vi "Wärmepumpe.ReadZustandsgrösse.vi"(0 "Wärmepumpe in":refnum<data-value>, 5 "error in":errorcluster) -> (11 "Verdichter 1":bool, 13 "Verdichter 2":bool, 14 "Wärmepumpe out":refnum<data-value>, 15 "Heizleistung [W]":dbl, 16 "Kälteleistung [W]":dbl, 17 "Vorlauftemperatur Heizkreislauf [°C]":dbl, 18 "Vorlauftemperatur Solekreislauf [°C]":dbl, 19 "error out":errorcluster)   [LabVIEW 2016, in "Wärmepumpe.lvclass"]
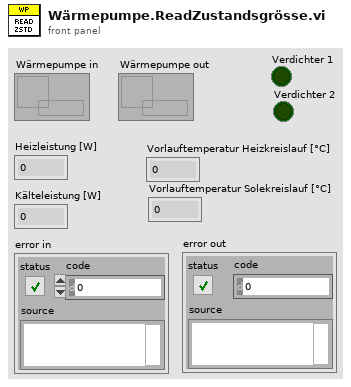
[diagram p1: front panel]
types:
  T1 = typedef "Wärmepumpe.lvclass/Wärmepumpe.Zustandsgrössen.ctl" = cluster{"Vorlauftemperatur Heizkreislauf[°C]":dbl, "Vorlauftemperatur Solekreislauf[°C]":dbl, "Heizleistung [W]":dbl, "Kälteleistung [W]":dbl, "Verdichter 1":bool, "Verdichter 2":bool}
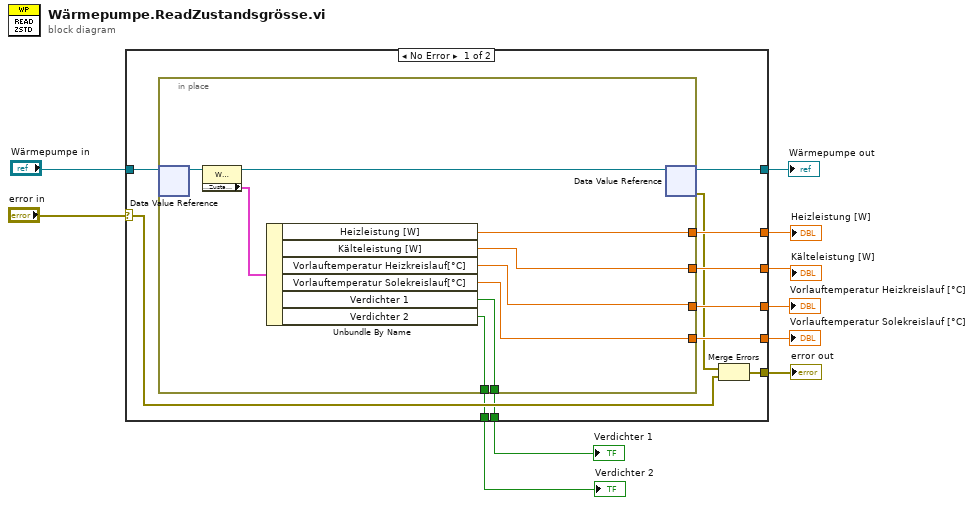
[diagram p0: block diagram]
diagram:
  n1 = case shown="No Error" "error in" {
    selector: "error in" -> [w15 w32]
    tunnel: "Wärmepumpe in" -> [w21 w31]
    tunnel: [w20 w31] -> w9
    tunnel: [w19 _] -> w8
    tunnel: [w18 _] -> w7
    tunnel: [w17 _] -> w6
    tunnel: [w16 _] -> w5
    tunnel: [w13 w32] -> w3
    tunnel: [w12 _] -> w2
    tunnel: [w11 _] -> w1
    frame No Error {
      n2 = in-place {
        in-place-border: [w28] -> w19
        in-place-border: [w27] -> w18
        in-place-border: [w25] -> w17
        in-place-border: [w24] -> w16
        in-place-border: [w23] -> w12
        in-place-border: [w22] -> w11
        n3 = in-place-dvr #1(w21) -> (w30:refnum<class "Wärmepumpe.lvclass">)  [unwired: 1 out]
        n4 = property class="Wärmepumpe.lvclass"(reference=w30) -> (reference out=w29:refnum<class "Wärmepumpe.lvclass">, "Accessors:Wärmepumpe.Zustandsgrössen"=w26:T1)  [unwired: 1 in, 1 out]
        n5 = Unbundle By Name(w26) -> ("Heizleistung [W]"=w28:dbl, "Kälteleistung [W]"=w27:dbl, "Vorlauftemperatur Heizkreislauf[°C]"=w25:dbl, "Vorlauftemperatur Solekreislauf[°C]"=w24:dbl, "Verdichter 1"=w23:bool, "Verdichter 2"=w22:bool)
        n6 = in-place-dvr #1(w29) -> (w20:refnum<data-value>, w14:errorcluster)
      }
      n7 = Merge Errors(w14, w15) -> (w13:errorcluster)
    }
    frame Error {
    }
  }
  "Heizleistung [W]" <- w8
  "Kälteleistung [W]" <- w7
  "Wärmepumpe out" <- w9
  "Vorlauftemperatur Heizkreislauf [°C]" <- w6
  "Vorlauftemperatur Solekreislauf [°C]" <- w5
  "error out" <- w3
  "Verdichter 1" <- w2
  "Verdichter 2" <- w1
